vi "Verify XNET Sessions.vi"(8 "error in (no error)":errorcluster, 11 "XNET Sessions":cluster{refnum<k21>[], "Address":u8}[](array[cluster])) -> (0 "error out":errorcluster)   [LabVIEW 2021, in "J1939-22_Engine.lvclass"]
uses:
  J1939-22_Engine.lvclass
  <resource>/objmgr/xnet.rc
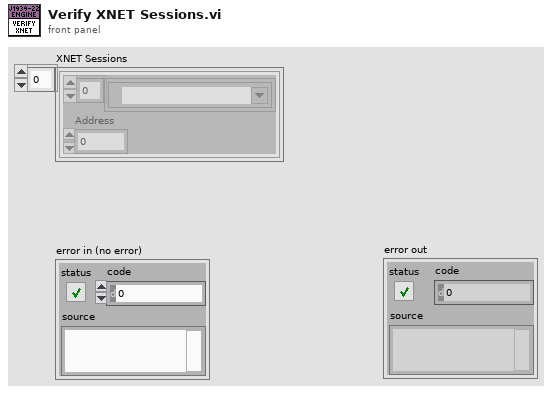
[diagram p1: front panel]
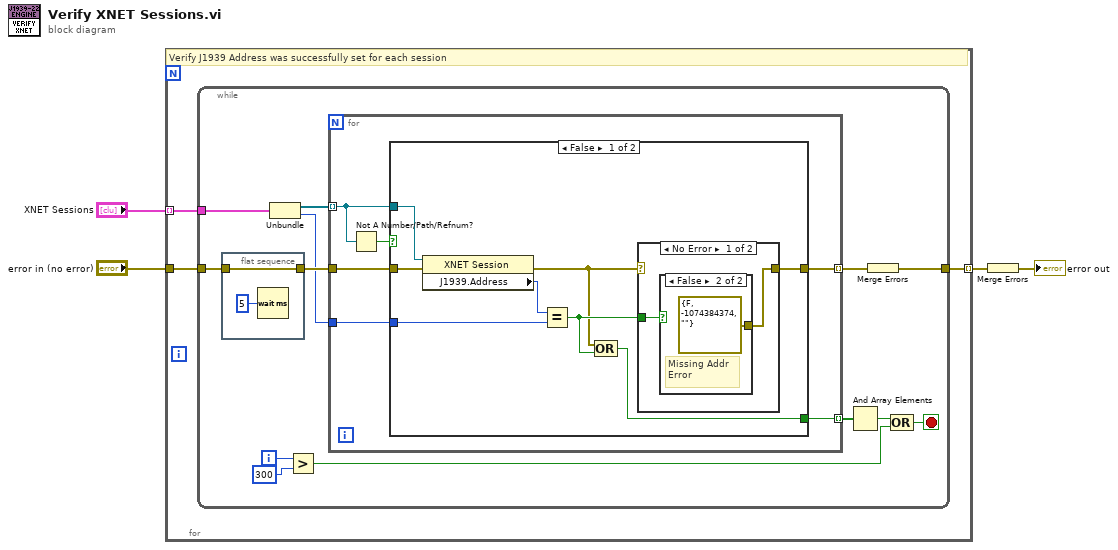
[diagram p0: block diagram]
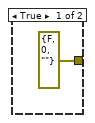
[diagram p2: hidden frame]
diagram:
  n1 = for {
    tunnel: "error in (no error)" -> [w7]
    tunnel: [w6] -> w2 mode=indexing
    tunnel: "XNET Sessions" -> [w5] mode=indexing
    # "Verify J1939 Address was successfully set for each session"
    n2 = while {
      tunnel: w7 -> [w17]
      tunnel: [w19] -> w6
      tunnel: w5 -> [w10]
      i -> [w15]
      stop <- w11 stop-if-true
      n3 = flat-sequence {
        tunnel: [w22] -> w18
        tunnel: w17 -> [w22]
        frame #0 {
          n4 = Wait (ms)(milliseconds to wait=u32 5) -> ()  [unwired: 1 out]
        }
      }
      n5 = Unbundle(w10) -> (w8:refnum<k21>[], "Address"=w9:u8)
      n6 = Greater?(x=w15, y=300) -> (0:w12:bool)
      n7 = for {
        tunnel: w18 -> [w28]
        tunnel: [w27] -> w20 mode=indexing
        tunnel: w8 -> [w26] mode=indexing
        tunnel: w9 -> [w24]
        tunnel: [w23] -> w14 mode=indexing
        n8 = Not A Number/Path/Refnum?(number/path/refnum=w26) -> (NaN/Path/Refnum?=w25:bool)
        n9 = case shown="False" w25 {
          selector: w25 -> [_ w42]
          tunnel: w28 -> [w34 w43]
          tunnel: [w33 w43] -> w27
          tunnel: w26 -> [w31 _]
          tunnel: w24 -> [w32 _]
          tunnel: [w29 w42] -> w23
          frame False {
            n10 = property class="XNET Session"(reference=w31, error in=w34) -> (error out=w35:errorcluster, "J1939.Address"=w30:u8)  [unwired: 1 out]
            n11 = Equal?(x=w30, y=w32) -> (x = y?=w36:bool)
            n12 = Compound Arithmetic op=OR(w35, w36) -> (w29:bool)
            n13 = case shown="No Error" w35 {
              selector: w35 -> [_ w41]
              tunnel: w36 -> [w38 _]
              tunnel: [w37 w41] -> w33
              frame No Error {
                n14 = case shown="False" w38 {
                  tunnel: [errorcluster {"status"=FALSE, "code"=0, "source"=""} ("error out") errorcluster {"status"=FALSE, "code"=-1074384374, "source"=""} ("error out")] -> w37
                  frame True {
                  }
                  frame False {
                    # "Missing Addr\nError"
                  }
                }
              }
              frame Error {
              }
            }
          }
          frame True {
          }
        }
      }
      n15 = And Array Elements(Boolean array=w14) -> (logical AND=w13:bool)
      n16 = Merge Errors(w20) -> (w19:errorcluster)
      n17 = Compound Arithmetic op=OR(w13, w12) -> (w11:bool)
    }
  }
  n18 = Merge Errors(w2) -> (→"error out":errorcluster)
